vi "ServiceModeTest0.vi"(0 "GEA2 Reference In":refnum<k24>, 2 "ON Erd_UiLedBitmap Value":string="0F", 3 "OFF Erd_UiLedBitmap Value":string="00", 5 "MC GEA Inputs":T3={"Source"=228, "Destination"=36} {"Destination" format="%.0x"; "Source" format="%.0x"}, 7 "UI GEA Inputs":T3={"Source"=228, "Destination"=37} {"Destination" format="%.0x"; "Source" format="%.0x"}, 11 "Error In":errorcluster, 12 "Board Index":i32, 13 "Loop Rate (ms)":u32=250, 14 "Timeout (s)":dbl=5.0 format="%#_13g") -> (4 "GEA2 Reference Out":refnum<k24>, 6 "Pass/Fail?":bool, 8 "Report Text":string, 15 "Error Out":errorcluster)   [LabVIEW 2016]
uses:
  Q:/Common/DLLs/GEA3/GeaCommunication.dll
  Common/DLLs/GEA3/GeaCommunication.dll
  Common/LabVIEW GEA2 Toolkit/LabVIEW_GEA2_Toolkit.lvlibp/type defs/Source_Destination.ctl
  Common/LabVIEW GEA2 Toolkit/LabVIEW_GEA2_Toolkit.lvlibp/type defs/ERD Read Data In.ctl
  Common/LabVIEW GEA2 Toolkit/LabVIEW_GEA2_Toolkit.lvlibp/type defs/Data Type.ctl
  Common/Type Defs/JL_Buttons.ctl
  Common/LabVIEW GEA2 Toolkit/LabVIEW_GEA2_Toolkit.lvlibp
panel:
  in  "Erd_PlayTuneId ERD Number":T1[](array[typedef])=[{"ERD Number"=61443, "Data Type"=enum."string"}] {"ERD Number" format="%.0x"}
  in  "Erd_UiLedBitmap ERD Number":T1={"ERD Number"=61729, "Data Type"=enum."string"} {"ERD Number" format="%.0x"}
  # "Suggested to keep values as default\nunless something changes in the future"
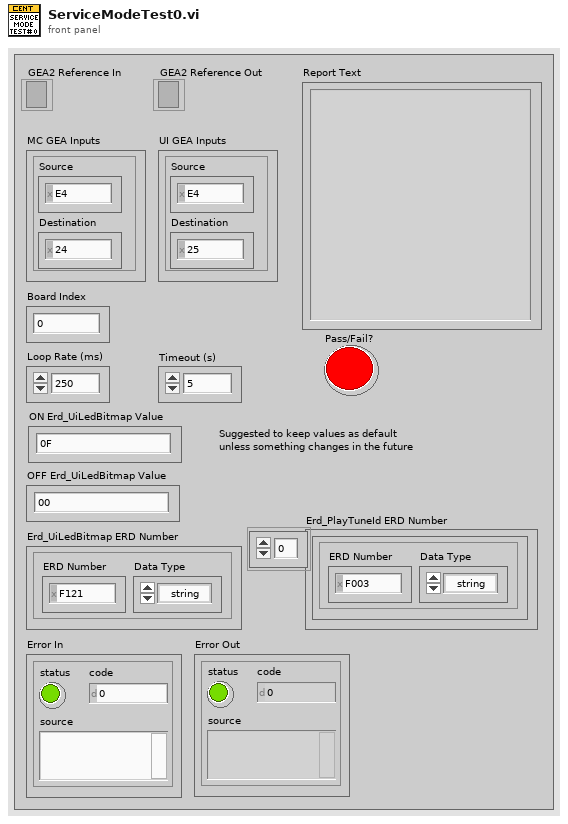
[diagram p1: front panel]
types:
  T1 = typedef "LabVIEW_GEA2_Toolkit.lvlibp/ERD Read Data In.ctl" = cluster{"ERD Number":u16, "Data Type":T2}
  T2 = typedef "LabVIEW_GEA2_Toolkit.lvlibp/Data Type.ctl" = enum16{"string", "boolean", "uint8_t", "uint16_t", "uint32_t", "uint64_t", "int8_t", "int16_t", "int32_t", "int64_t"}
  T3 = typedef "LabVIEW_GEA2_Toolkit.lvlibp/Source_Destination.ctl" = cluster{"Source":u8, "Destination":u8}
  T4 = enum16{"EQ (==)", "NE (!=)", "GT (>)", "LT (<)", "GE (>=)", "LE (<=)", "GTLT(> <)", "GELE (>= <=)", "GELT (>= <)", "GTLE (> <=)", "LTGT (< >)", "LEGE (<= >=)", "LEGT (<= >)", "LTGE (< >=)", "No Comparison"}
  T5 = typedef "JL_Buttons.ctl" = enum16{"Power", "Start / Pause ", "Temp Option ", "Dryness Level", "Time Option", "Time Increment ", "Time Decrement ", "MyCycle", "eDry ", "Delay", "Extended Tumble", "Control Lock", "Volume/Signal", "Damp Alert / Drum Light", "Unused", "(SW213)", "(SW322)", "Clear / Reset"}
  T6 = typedef "LabVIEW_GEA2_Toolkit.lvlibp/ERD Read Data Out.ctl" = cluster{"ERD Number":u16, "Data":string}
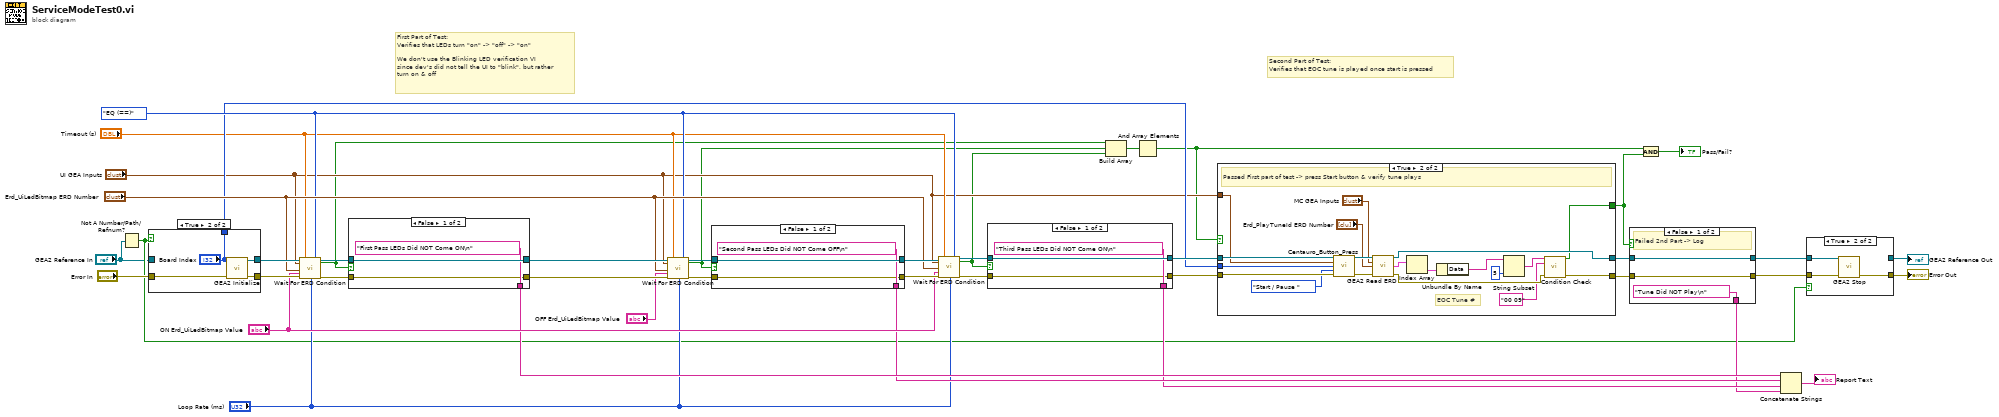
[diagram p0: block diagram]
diagram:
  w25 = T4."EQ (==)" ("Comparison")
  # "Second Part of Test:\nVerifies that EOC tune is played once start is pressed"
  # "First Part of Test:\nVerifies that LEDs turn \"on\" -> \"off\" -> \"on\"\n\nWe don't use the Blinking LED verification VI\nsince dev's did not tell the UI to \"blink\", but rather\nturn on & off"
  n1 = Not A Number/Path/Refnum?(number/path/refnum="GEA2 Reference In") -> (NaN/Path/Refnum?=w2:bool)
  n2 = case shown="True" w2 {
    tunnel: [w44 w49] -> w41
    tunnel: "Error In" -> [w44 w48]
    tunnel: [w45 w47] -> w42
    tunnel: "GEA2 Reference In" -> [w45 _]
    tunnel: [_ "Board Index"] -> w19
    frame False {
    }
    frame True {
      n3 = call "GEA2 Initialize.vi"("Board Index"="Board Index", "error in"=w48) -> ("GEA2 Reference Out"=w47:refnum<k24>, "error out"=w49:errorcluster)  [unwired: 11 in, 1 out]
    }
  }
  n4 = call "Wait For ERD Condition.vi"("GEA2 Reference In"=w42, "GEA Inputs"="UI GEA Inputs", "ERD Read Data"="Erd_UiLedBitmap ERD Number", "Expected Low"="ON Erd_UiLedBitmap Value", "Error In"=w41, "Timeout (s)"="Timeout (s)", "Loop Rate (ms)"="Loop Rate (ms)", "Comparison"=w25) -> ("GEA2 Reference Out"=w40:refnum<k24>, "Pass/Fail?"=w7:bool, "Error Out"=w39:errorcluster)  [unwired: 7 in, 2 out]
  n5 = case shown="False" w7 {
    tunnel: w40 -> [w52 w53]
    tunnel: w39 -> [w50 w54]
    tunnel: [w50 w54] -> w37
    tunnel: [w52 w53] -> w38
    tunnel: ["First Pass LEDs Did NOT Come ON\n" _] -> w26
    frame False {
    }
    frame True {
    }
  }
  n6 = call "Wait For ERD Condition.vi"("GEA2 Reference In"=w38, "GEA Inputs"="UI GEA Inputs", "ERD Read Data"="Erd_UiLedBitmap ERD Number", "Expected Low"="OFF Erd_UiLedBitmap Value", "Error In"=w37, "Timeout (s)"="Timeout (s)", "Loop Rate (ms)"="Loop Rate (ms)", "Comparison"=w25) -> ("GEA2 Reference Out"=w35:refnum<k24>, "Pass/Fail?"=w6:bool, "Error Out"=w34:errorcluster)  [unwired: 7 in, 2 out]
  n7 = case shown="False" w6 {
    tunnel: w35 -> [w57 w58]
    tunnel: w34 -> [w55 w59]
    tunnel: [w55 w59] -> w29
    tunnel: [w57 w58] -> w30
    tunnel: ["Second Pass LEDs Did NOT Come OFF\n" _] -> w24
    frame False {
    }
    frame True {
    }
  }
  n8 = call "Wait For ERD Condition.vi"("GEA2 Reference In"=w30, "GEA Inputs"="UI GEA Inputs", "ERD Read Data"="Erd_UiLedBitmap ERD Number", "Expected Low"="ON Erd_UiLedBitmap Value", "Error In"=w29, "Timeout (s)"="Timeout (s)", "Loop Rate (ms)"="Loop Rate (ms)", "Comparison"=w25) -> ("GEA2 Reference Out"=w32:refnum<k24>, "Pass/Fail?"=w5:bool, "Error Out"=w31:errorcluster)  [unwired: 7 in, 2 out]
  n9 = case shown="False" w5 {
    tunnel: w32 -> [w62 w63]
    tunnel: w31 -> [w60 w64]
    tunnel: [w60 w64] -> w21
    tunnel: [w62 w63] -> w22
    tunnel: ["Third Pass LEDs Did NOT Come ON\n" _] -> w23
    frame False {
    }
    frame True {
    }
  }
  n10 = Build Array(w7, w6, w5) -> (w4:bool[])
  n11 = And Array Elements(Boolean array=w4) -> (logical AND=w3:bool)
  n12 = case shown="True" w3 {
    selector: w3 -> [w65 _]
    tunnel: w22 -> [w67 w86]
    tunnel: w21 -> [w66 w85]
    tunnel: [w67 w74] -> w13
    tunnel: [w66 w73] -> w11
    tunnel: w19 -> [_ w84]
    tunnel: [w65 w72] -> w15
    tunnel: "UI GEA Inputs" -> [_ w71]
    frame False {
      # "Failed first part of test -> do nothing"
    }
    frame True {
      # "EOC Tune #"
      # "Passed First part of test -> press Start button & verify tune plays"
      n13 = call "Centauro_Button_Press.vi"("GEA2 Reference In"=w86, "GEA Inputs"=w71, "Board Index"=w84, "Button"=JL_Buttons."Start / Pause ", "Error In"=w85) -> ("GEA2 Reference Out"=w82:refnum<k24>, "Error Out"=w81:errorcluster)  [unwired: 9 in]
      n14 = call "GEA2 Read ERD.vi"("GEA2 Reference In"=w82, "GEA Inputs"="MC GEA Inputs", "Read ERD List"="Erd_PlayTuneId ERD Number", "Error In"=w81) -> ("GEA2 Reference Out"=w74:refnum<k24>, "ERD Data Out"=w70:T6[], "Error Out"=w76:errorcluster)  [unwired: 8 in, 1 out]
      n15 = Index Array(array=w70) -> (element=w69:T6)  [unwired: 1 in]
      n16 = Unbundle By Name(w69) -> ("Data"=w68:string)
      n17 = String Subset(string=w68, length (rest)=5 ("length (rest)")) -> (substring=w77:string)  [unwired: 1 in]
      n18 = call "Condition Check.vi"("Actual"=w77, "Low"="00 09", "Error In"=w76) -> ("Pass/Fail"=w72:bool, "Error Out"=w73:errorcluster)  [unwired: 10 in, 1 out]
    }
  }
  n19 = case shown="False" w15 {
    tunnel: ["Tune Did NOT Play\n" _] -> w14
    tunnel: [w88 w91] -> w12
    tunnel: w13 -> [w88 w91]
    tunnel: [w87 w90] -> w10
    tunnel: w11 -> [w87 w90]
    frame False {
      # "Failed 2nd Part -> Log"
    }
    frame True {
      # "Passed 2nd Part -> Do Nothing"
    }
  }
  n20 = And(x=w3, y=w15) -> (x .and. y?=→"Pass/Fail?":bool)
  n21 = Concatenate Strings(w26, w24, w23, w14) -> (→"Report Text":string)
  n22 = case shown="True" w2 {
    tunnel: [w92 w96] -> w20
    tunnel: w12 -> [w93 w95]
    tunnel: w10 -> [w92 w94]
    tunnel: [w93 _] -> w9
    frame False {
    }
    frame True {
      n23 = call "GEA2 Stop.vi"("GEA2 Reference In"=w95, "Error In"=w94) -> ("Error Out"=w96:errorcluster)  [unwired: 13 in]
    }
  }
  "GEA2 Reference Out" <- w9
  "Error Out" <- w20
